vi "Protection_DSP.vi"(8 "error in (no error)":errorcluster caption="에러 입력(에러 없음)", 9 "OCP Level":dbl, 10 "OVP Level":dbl, 11 "VISA resource name":refnum<visa-resource-name>) -> (0 "error out":errorcluster caption="에러 출력", 3 "VISA resource name Out":refnum<visa-resource-name>)   [LabVIEW 2019]
uses:
  b59ef056-d11c-42a8-9a9f-ec81e679a916.vi
  SubVIs/common/Glob_Ref.vi
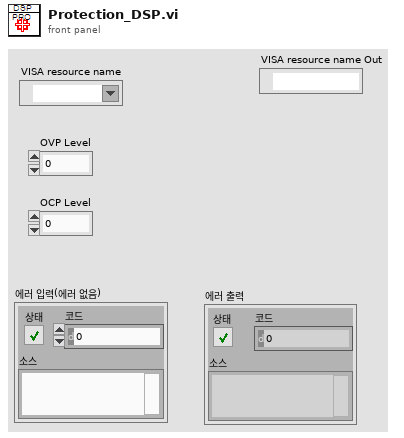
[diagram p1: front panel]
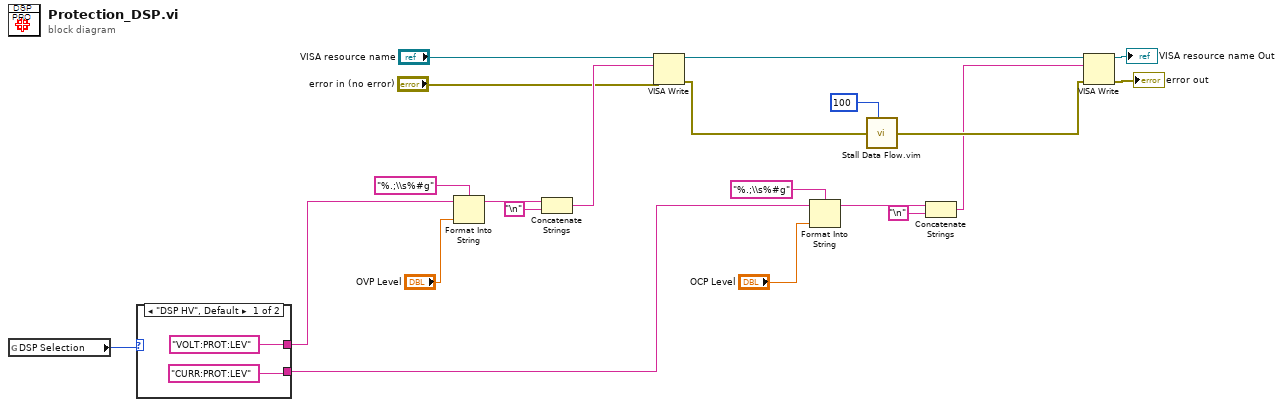
[diagram p0: block diagram]
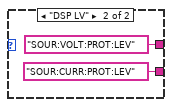
[diagram p2: hidden frame]
diagram:
  n1 = global read "Glob_Ref.vi" "DSP Selection"() -> (w3:enum32{"DSP HV", "DSP LV"})
  n2 = case shown="\"DSP HV\", Default" w3 {
    tunnel: ["VOLT:PROT:LEV" "SOUR:VOLT:PROT:LEV"] -> w2
    tunnel: ["CURR:PROT:LEV" "SOUR:CURR:PROT:LEV"] -> w1
    frame "DSP HV", Default {
    }
    frame "DSP LV" {
    }
  }
  n3 = Format Into String(format string="%.;\\s%#g", initial string=w2, "OVP Level") -> (resulting string=w12:string)  [unwired: 1 in, 1 out]
  n4 = Concatenate Strings(w12, "\n") -> (w11:string)
  n5 = VISA Write(VISA resource name="VISA resource name", write buffer=w11, error in (no error)="error in (no error)") -> (VISA resource name out=w6:refnum<visa-resource-name>, error out=w7:errorcluster)  [unwired: 1 out]
  n6 = Format Into String(format string="%.;\\s%#g", initial string=w1, "OCP Level") -> (resulting string=w10:string)  [unwired: 1 in, 1 out]
  n7 = call "Stall Data Flow.vim"("value in"=w7, "milliseconds to wait"=u32 100) -> ("value out"=w5:errorcluster)  [unwired: 1 out]
  n8 = Concatenate Strings(w10, "\n") -> (w4:string)
  n9 = VISA Write(VISA resource name=w6, write buffer=w4, error in (no error)=w5) -> (VISA resource name out=→"VISA resource name Out":refnum<visa-resource-name>, error out=→"error out":errorcluster)  [unwired: 1 out]
